vi "AssetMgrGetMissingChannelsFromHardwareResponse_Parse.vi"(8 "error in (no error)":errorcluster, 11 "Message":T6) -> (0 "error out":errorcluster, 1 "Body":T1, 2 "Header":T5, 3 "AssetMgrGetMissingChannelsFromHardwareResponse":T4)   [LabVIEW 2017]
uses:
  <vilib>/addons/InsightCM/MessageBus/Base/controls/Message.ctl
  <vilib>/addons/InsightCM/MessageBus/Base/controls/MessageHeader.ctl
  <vilib>/addons/InsightCM/MessageBus/Base/controls/KeyValuePair.ctl
  <vilib>/addons/InsightCM/MessageBus/MessageLibrary/AssetManager/controls/AssetMgrGetMissingChannelsFromHardwareResponse.ctl
  <vilib>/addons/InsightCM/MessageBus/MessageLibrary/AssetManager/controls/AssetMgrGetMissingChannelsFromHardwareResponseBody.ctl
  <vilib>/addons/InsightCM/MessageBus/Base/controls/Channel.ctl
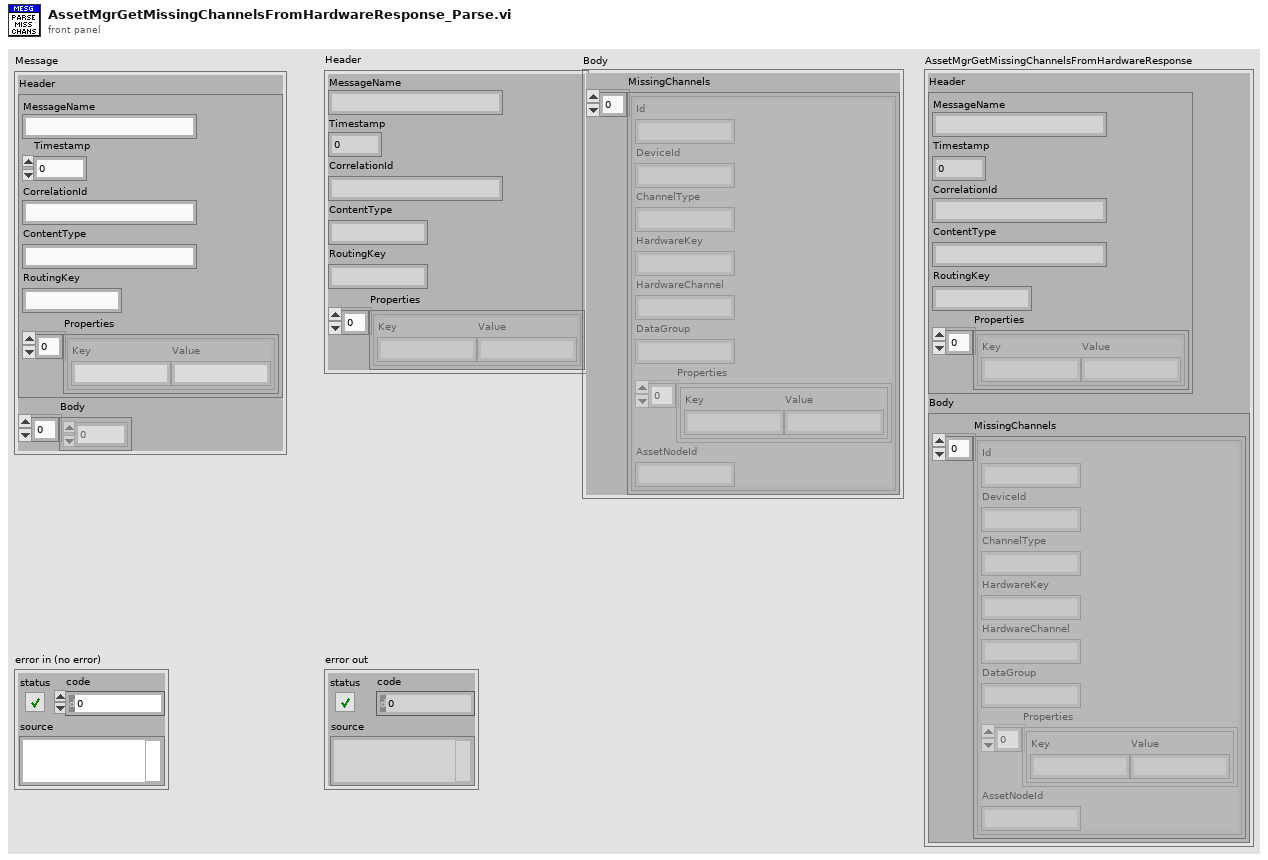
[diagram p1: front panel]
types:
  T1 = typedef "AssetMgrGetMissingChannelsFromHardwareResponseBody.ctl" = cluster{"MissingChannels":T2[]}
  T2 = typedef "Channel.ctl" = cluster{"Id":string, "DeviceId":string, "ChannelType":string, "HardwareKey":string, "HardwareChannel":string, "DataGroup":string, "Properties":T3[], "AssetNodeId":string}
  T3 = typedef "KeyValuePair.ctl" = cluster{"Key":string, "Value":string}
  T4 = typedef "AssetMgrGetMissingChannelsFromHardwareResponse.ctl" = cluster{"Header":T5, "Body":T1}
  T5 = typedef "MessageHeader.ctl" = cluster{"MessageName":string, "Timestamp":i64, "CorrelationId":string, "ContentType":string, "RoutingKey":string, "Properties":T3[]}
  T6 = typedef "Message.ctl" = cluster{"Header":T5, "Body":u8[]}
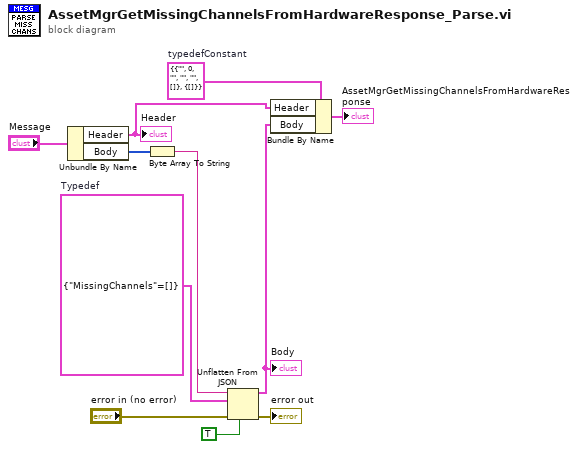
[diagram p0: block diagram]
diagram:
  w3 = T4 {"Header"={"MessageName"="", "Timestamp"=0, "CorrelationId"="", "ContentType"="", "RoutingKey"="", "Properties"=[]}, "Body"={"MissingChannels"=[]}}  # typedefConstant
  w7 = T1 {"MissingChannels"=[]}  # Typedef
  n1 = Unbundle By Name("Message") -> ("Header"=w9:T5, "Body"=w1:u8[])
  "Header" <- w9
  n2 = Byte Array To String(unsigned byte array=w1) -> (string=w6:string)
  n3 = Unflatten From JSON(JSON string=w6, type and defaults=w7, default null elements? (F)=TRUE, error in (no error)="error in (no error)") -> (value=w5:T1, error out=→"error out":errorcluster)  [unwired: 3 in]
  "Body" <- w5
  n4 = Bundle By Name(cluster=w3, "Header"=w9, "Body"=w5) -> (→"AssetMgrGetMissingChannelsFromHardwareResponse":T4)
